vi "Unregister.vi"(8 "error in (no error)":errorcluster, 11 "logger name":string) -> (0 "error out":errorcluster, 3 "logger":refnum<class "Logger.lvclass">)   [LabVIEW 2018, in "GLog.lvlib" / "Registry.lvlib"]
uses:
  Registry.lvlib
  Registry Actions.ctl
  api/logger_class/Logger.lvclass
  Utilities/Utilities.lvlib
panel:
  # "Connector Pane"
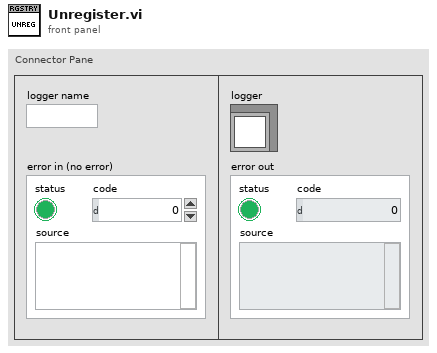
[diagram p1: front panel]
types:
  T1 = typedef "GLog.lvlib/Registry.lvlib/Registry Actions.ctl" = enum16{"Register", "Log", "Enable", "Enable All", "Disable", "Disable All", "List", "Unregister", "Unregister All"}
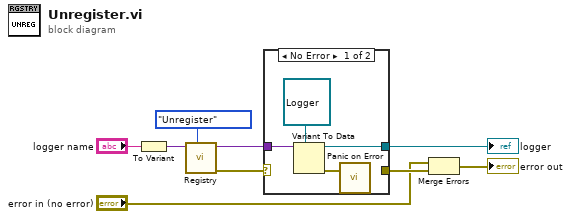
[diagram p0: block diagram]
diagram:
  n1 = To Variant(anything="logger name") -> (Variant=w6:variant)
  n2 = call "Registry.vi"("action"=Registry_Actions."Unregister", "data in"=w6) -> ("error out"=w3:errorcluster, "data out"=w4:variant)  [unwired: 8 in]
  n3 = case shown="No Error" w3 {
    selector: w3 -> [_ w14]
    tunnel: w4 -> [w13 _]
    tunnel: [w11 _] -> w8
    tunnel: [_ w14] -> w7
    frame No Error {
      n4 = Variant To Data(type=refnum<class "Logger.lvclass"> refnum ("Logging.lvlib:Logger.lvclass"), Variant=w13) -> (data=w11:refnum<class "Logger.lvclass">, error out=w10:errorcluster)  [unwired: 1 in]
      n5 = call "Panic on Error.vi"("error in (no error)"=w10) -> ()  [unwired: 3 in]
    }
    frame Error {
    }
  }
  "logger" <- w8
  n6 = Merge Errors("error in (no error)", w7) -> (→"error out":errorcluster)
